vi "init.vi"(8 "error in (no error)":errorcluster, 10 "Config":string, 11 "MOXAIP in":refnum<class "MOXAIP.lvclass">) -> (0 "error out":errorcluster, 3 "MOXAIP out":refnum<class "MOXAIP.lvclass">)   [LabVIEW 2015, in "Serializer.lvlib" / "MOXAIP.lvclass"]
uses:
  MOXAIP.lvclass
  MOXAIP.lvclass/MOXAIP.ctl
panel:
  # "ISA010"
  # "{\"IP\":\"192.168.20.118\",\"port\":4001}"
  # "{\"IP\":\"192.168.20.118\",\"port\":4001}"
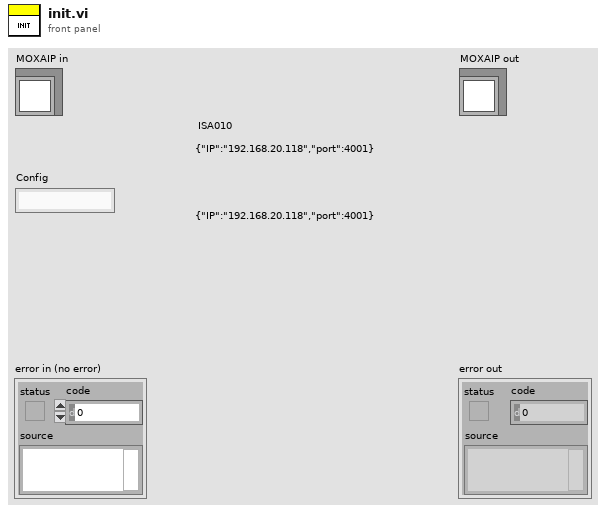
[diagram p1: front panel]
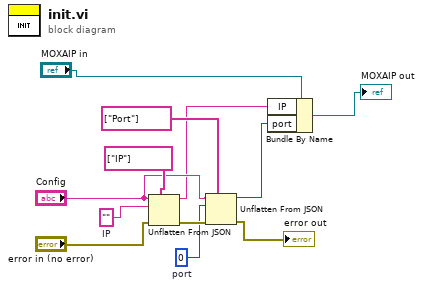
[diagram p0: block diagram]
diagram:
  w7 = u16 0  # port
  w8 = ""  # IP
  n1 = Unflatten From JSON(path=string[] ["IP"], JSON string="Config", type and defaults=w8, error in (no error)="error in (no error)") -> (value=w3:string, error out=w11:errorcluster)  [unwired: 3 in]
  n2 = Unflatten From JSON(path=string[] ["Port"], JSON string="Config", type and defaults=w7, error in (no error)=w11) -> (value=w2:u16, error out=→"error out":errorcluster)  [unwired: 3 in]
  n3 = Bundle By Name(cluster="MOXAIP in", "IP"=w3, "port"=w2) -> (→"MOXAIP out":refnum<class "MOXAIP.lvclass">)
